vi "InitClimber.vi"   [LabVIEW 2019]
uses:
  <vilib>/Rock Robotics/WPI/Solenoid/WPI_SolenoidOpenDouble.vi
  <vilib>/Rock Robotics/WPI/Solenoid/WPI_SolenoidChannel.ctl
  refnums.vi
types:
  T1 = typedef "WPI_SolenoidChannel.ctl" = enum8{"Solenoid 0", "Solenoid 1", "Solenoid 2", "Solenoid 3", "Solenoid 4", "Solenoid 5", "Solenoid 6", "Solenoid 7", "Invalid"}
  T2 = typedef "WPI_SolenoidDevRef.ctl" = cluster{"DevStatus":errorcluster, "Pneumatics Control Module":u8, "Forward Solenoid Channel":T1, "Reverse Solenoid Channel":T1}
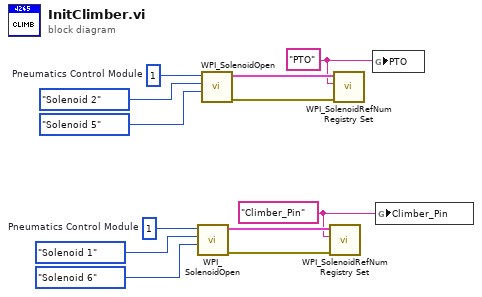
[diagram p0: block diagram]
diagram:
  w1 = "Climber_Pin" ("refnum name")
  w7 = u8 1  # Pneumatics Control Module
  w2 = "PTO" ("refnum name")
  w12 = u8 1  # Pneumatics Control Module
  n1 = call-poly <vilib>:"WPI_SolenoidOpen.vi"("Reverse Solenoid Channel"=WPI_SolenoidChannel."Solenoid 6", "Forward Solenoid Channel"=WPI_SolenoidChannel."Solenoid 1", "Pneumatics Control Module (0)"=w7) -> ("error out"=w3:errorcluster, "SolenoidDevRef"=w4:T2)  [unwired: 7 in]
  n2 = call-poly <vilib>:"WPI_SolenoidOpen.vi"("Reverse Solenoid Channel"=WPI_SolenoidChannel."Solenoid 5", "Forward Solenoid Channel"=WPI_SolenoidChannel."Solenoid 2", "Pneumatics Control Module (0)"=w12) -> ("error out"=w8:errorcluster, "SolenoidDevRef"=w9:T2)  [unwired: 7 in]
  n3 = call <vilib>:"WPI_SolenoidRefNum Registry Set.vi"("error in (no error)"=w3, "refnum name"=w1, "SolenoidDevRef"=w4) -> ()  [unwired: 7 in, 2 out]
  n4 = call <vilib>:"WPI_SolenoidRefNum Registry Set.vi"("error in (no error)"=w8, "refnum name"=w2, "SolenoidDevRef"=w9) -> ()  [unwired: 7 in, 2 out]
  n5 = global write "refnums.vi" "PTO"(w2) -> ()
  n6 = global write "refnums.vi" "Climber_Pin"(w1) -> ()
